vi "Build stringplusnum substring.vi"(1 "Sequence":u16(ring) items=["String1String2String3Value1Value2", "String1String2Value1String3Value2"], 2 "String1":string[](array[string]), 3 "String2":string[](array[string]), 4 "String3":string[](array[string]), 5 "error in":errorcluster, 6 "Value1":dbl[](array[numeric]) format="%.6f", 7 "Value2":dbl[](array[numeric]) format="%.6f", 8 "No.of digits Val1":i16=6, 9 "No.of digits Val2":i16=6, 10 "Input selection":T1={"With string1?"=TRUE, "With string2?"=TRUE, "With string3?"=TRUE, "With value1?"=TRUE, "With value2?"=FALSE}) -> (14 "Substring":string, 19 "error out":errorcluster)   [LabVIEW 2020]
doc: "This VI builds a command substring by combining up to three strings and two values. Sub-VI for FCG.vi, CTC.vi and DAS.vi"
panel:
  # "This vi builds a command substring by combining up to three strings and two values."
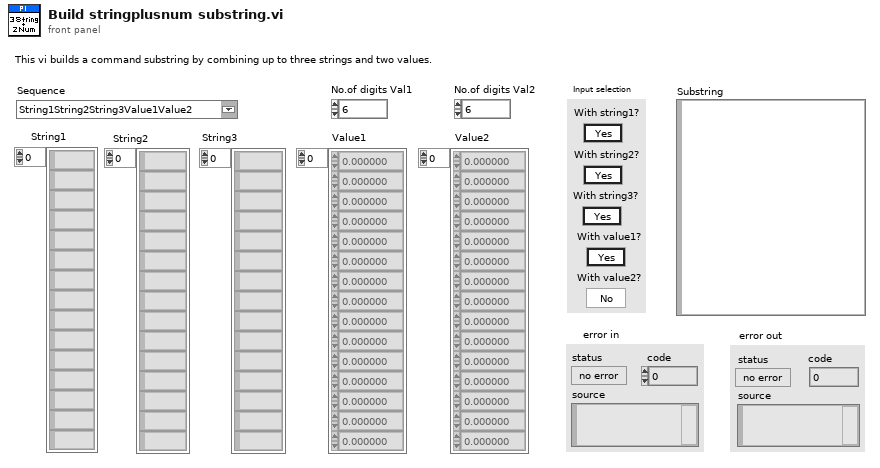
[diagram p1: front panel]
types:
  T1 = cluster{"With string1?":bool, "With string2?":bool, "With string3?":bool, "With value1?":bool, "With value2?":bool}
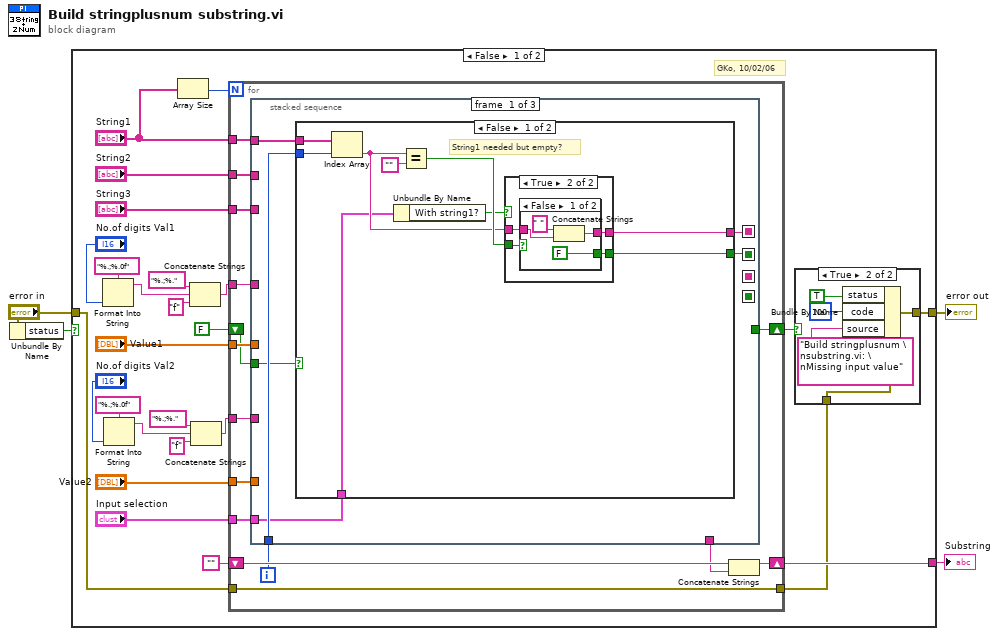
[diagram p0: block diagram]
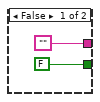
[diagram p3: hidden frame]
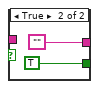
[diagram p4: hidden frame]
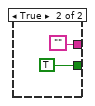
[diagram p5: hidden frame]
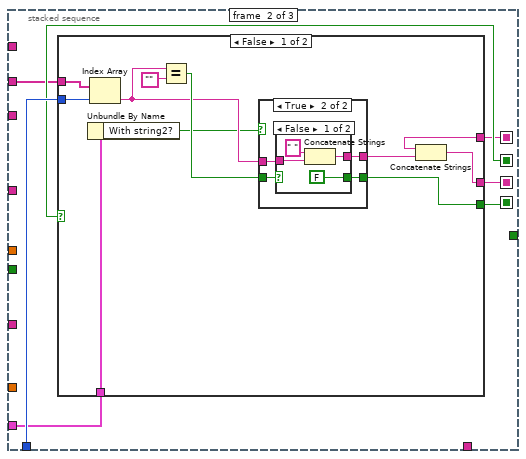
[diagram p6: hidden frame]
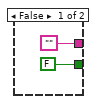
[diagram p7: hidden frame]
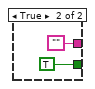
[diagram p8: hidden frame]
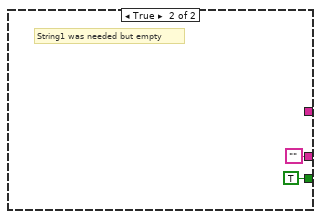
[diagram p9: hidden frame]
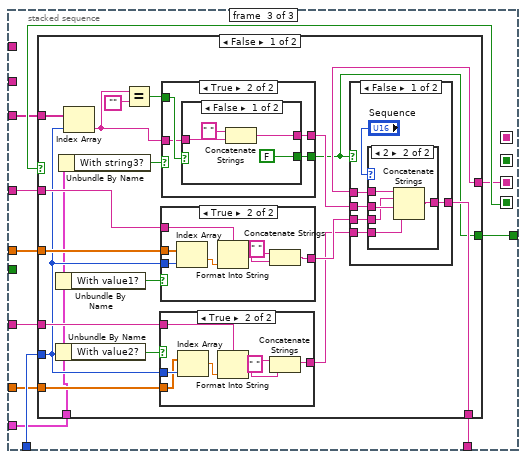
[diagram p10: hidden frame]
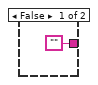
[diagram p11: hidden frame]
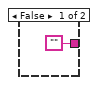
[diagram p12: hidden frame]
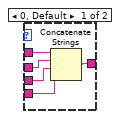
[diagram p13: hidden frame]
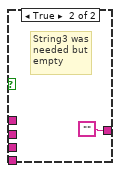
[diagram p14: hidden frame]
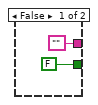
[diagram p15: hidden frame]
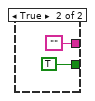
[diagram p16: hidden frame]
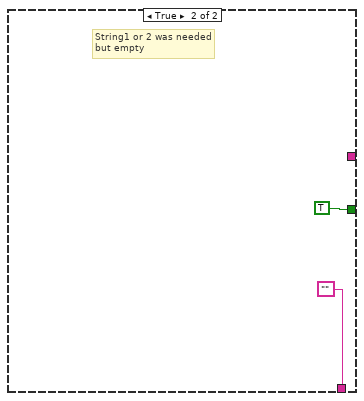
[diagram p17: hidden frame]
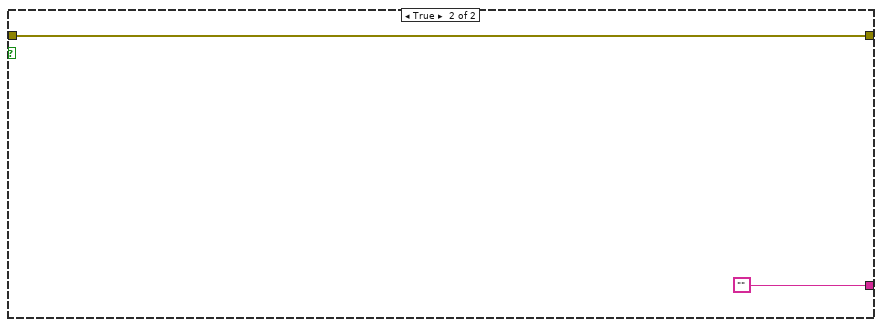
[diagram p18: hidden frame]
diagram:
  n1 = Unbundle By Name("error in") -> ("status"=w3:bool)
  n2 = case shown="False" w3 {
    tunnel: [w30 ""] -> w4
    tunnel: "error in" -> [w21 w190]
    tunnel: [w18 w190] -> w1
    frame False {
      # "GKo, 10/02/06"
      n3 = Format Into String(format string="%.;%.0f" ("Format String"), "No.of digits Val1") -> (resulting string=w13:string)  [unwired: 2 in, 1 out]
      n4 = Format Into String(format string="%.;%.0f" ("Format String"), "No.of digits Val2") -> (resulting string=w7:string)  [unwired: 2 in, 1 out]
      n5 = Array Size(array="String1") -> (size(s)=w28:i32)
      n6 = Concatenate Strings("%.;%." ("Format String"), w13, "f" ("Format String")) -> (w12:string)
      n7 = Concatenate Strings("%.;%." ("Format String"), w7, "f" ("Format String")) -> (w6:string)
      n8 = for {
        N: w28 -> [_]
        shift-right: [w50] -> w30
        shift-left: "" -> [w51]
        tunnel: "String1" -> [w48]
        tunnel: "String2" -> [w47]
        tunnel: "Value1" -> [w46]
        tunnel: w6 -> [w45]
        tunnel: "String3" -> [w44]
        tunnel: w12 -> [w42]
        tunnel: "Value2" -> [w41]
        shift-right: [w40] -> w20
        shift-left: FALSE -> [w39]
        tunnel: [w38] -> w19
        tunnel: w21 -> [w38]
        tunnel: "Input selection" -> [w37]
        i -> [w49]
        n9 = stacked-sequence {
          seq-local: [w55 _ _] -> [_ w82 _]
          seq-local: [w54 _ _] -> [_ w86 _]
          seq-local: [_ w85 _] -> [_ _ w120]
          seq-local: [_ w83 _] -> [_ _ w123]
          tunnel: w49 -> [w57 w87 w116]
          tunnel: w48 -> [w56 _ _]
          tunnel: w47 -> [_ w84 _]
          tunnel: w46 -> [_ _ w118]
          tunnel: w45 -> [_ _ w117]
          tunnel: w44 -> [_ _ w122]
          tunnel: [_ _ w121] -> w43
          tunnel: w42 -> [_ _ w119]
          tunnel: w41 -> [_ _ w115]
          tunnel: [_ _ w114] -> w40
          tunnel: w39 -> [w53 _ _]
          tunnel: w37 -> [w52 w81 w113]
          frame #0 {
            n10 = case shown="False" w53 {
              tunnel: w57 -> [w66 _]
              tunnel: w56 -> [w65 _]
              tunnel: [w61 ""] -> w55
              tunnel: [w60 TRUE] -> w54
              tunnel: w52 -> [w59 _]
              frame False {
                # "String1 needed but empty?"
                n11 = Index Array(array=w65, index=w66) -> (element=w62:string)
                n12 = Unbundle By Name(w59) -> ("With string1?"=w58:bool)
                n13 = Equal?(x=w62, y="") -> (x = y?=w63:bool)
                n14 = case shown="True" w58 {
                  tunnel: w63 -> [_ w72]
                  tunnel: ["" w71] -> w61
                  tunnel: [FALSE w70] -> w60
                  tunnel: w62 -> [_ w69]
                  frame False {
                  }
                  frame True {
                    n15 = case shown="False" w72 {
                      tunnel: [w73 ""] -> w71
                      tunnel: [FALSE TRUE] -> w70
                      tunnel: w69 -> [w75 _]
                      frame False {
                        n16 = Concatenate Strings(" " ("Substring"), w75) -> (w73:string)
                      }
                      frame True {
                      }
                    }
                  }
                }
              }
              frame True {
              }
            }
          }
          frame #1 {
            n17 = case shown="False" w86 {
              tunnel: w87 -> [w98 _]
              tunnel: [w92 ""] -> w85
              tunnel: w84 -> [w96 _]
              tunnel: [w93 TRUE] -> w83
              tunnel: w82 -> [w90 _]
              tunnel: w81 -> [w89 _]
              frame False {
                n18 = Unbundle By Name(w89) -> ("With string2?"=w88:bool)
                n19 = Index Array(array=w96, index=w98) -> (element=w94:string)
                n20 = Equal?(x=w94, y="") -> (x = y?=w95:bool)
                n21 = case shown="True" w88 {
                  tunnel: w95 -> [_ w104]
                  tunnel: ["" w103] -> w91
                  tunnel: [FALSE w102] -> w93
                  tunnel: w94 -> [_ w101]
                  frame False {
                  }
                  frame True {
                    n22 = case shown="False" w104 {
                      tunnel: [w107 ""] -> w103
                      tunnel: [FALSE TRUE] -> w102
                      tunnel: w101 -> [w105 _]
                      frame False {
                        n23 = Concatenate Strings(" " ("Substring"), w105) -> (w107:string)
                      }
                      frame True {
                      }
                    }
                  }
                }
                n24 = Concatenate Strings(w90, w91) -> (w92:string)
              }
              frame True {
                # "String1 was needed but empty"
              }
            }
          }
          frame #2 {
            n25 = case shown="False" w123 {
              tunnel: [w138 ""] -> w121
              tunnel: w122 -> [w142 _]
              tunnel: w120 -> [w125 _]
              tunnel: w119 -> [w136 _]
              tunnel: w118 -> [w135 _]
              tunnel: w117 -> [w134 _]
              tunnel: w116 -> [w133 _]
              tunnel: w115 -> [w132 _]
              tunnel: [w124 TRUE] -> w114
              tunnel: w113 -> [w129 _]
              frame False {
                n26 = Unbundle By Name(w129) -> ("With value1?"=w127:bool)
                n27 = Unbundle By Name(w129) -> ("With value2?"=w126:bool)
                n28 = Unbundle By Name(w129) -> ("With string3?"=w128:bool)
                n29 = Index Array(array=w142, index=w133) -> (element=w139:string)
                n30 = Equal?(x=w139, y="") -> (x = y?=w140:bool)
                n31 = case shown="True" w126 {
                  tunnel: w134 -> [_ w147]
                  tunnel: w133 -> [_ w146]
                  tunnel: ["" w145] -> w130
                  tunnel: w132 -> [_ w144]
                  frame False {
                  }
                  frame True {
                    n32 = Index Array(array=w144, index=w146) -> (element=w150:dbl)
                    n33 = Format Into String(format string=w147, w150) -> (resulting string=w148:string)  [unwired: 2 in, 1 out]
                    n34 = Concatenate Strings(" " ("Substring"), w148) -> (w145:string)
                  }
                }
                n35 = case shown="True" w127 {
                  tunnel: w136 -> [_ w155]
                  tunnel: w133 -> [_ w154]
                  tunnel: ["" w153] -> w131
                  tunnel: w135 -> [_ w152]
                  frame False {
                  }
                  frame True {
                    n36 = Index Array(array=w152, index=w154) -> (element=w158:dbl)
                    n37 = Format Into String(format string=w155, w158) -> (resulting string=w156:string)  [unwired: 2 in, 1 out]
                    n38 = Concatenate Strings(" " ("Substring"), w156) -> (w153:string)
                  }
                }
                n39 = case shown="True" w128 {
                  tunnel: w140 -> [_ w181]
                  tunnel: ["" w180] -> w137
                  tunnel: [FALSE w179] -> w124
                  tunnel: w139 -> [_ w178]
                  frame False {
                  }
                  frame True {
                    n40 = case shown="False" w181 {
                      tunnel: [w184 ""] -> w180
                      tunnel: [FALSE TRUE] -> w179
                      tunnel: w178 -> [w182 _]
                      frame False {
                        n41 = Concatenate Strings(" " ("Substring"), w182) -> (w184:string)
                      }
                      frame True {
                      }
                    }
                  }
                }
                n42 = case shown="False" w124 {
                  tunnel: [w163 ""] -> w138
                  tunnel: w125 -> [w162 _]
                  tunnel: w137 -> [w161 _]
                  tunnel: w131 -> [w160 _]
                  tunnel: w130 -> [w159 _]
                  frame False {
                    n43 = case shown="2" "Sequence" {
                      tunnel: [w169 w174] -> w163
                      tunnel: w162 -> [w168 w173]
                      tunnel: w161 -> [w167 w172]
                      tunnel: w160 -> [w166 w171]
                      tunnel: w159 -> [w165 w170]
                      frame 0, Default {
                        n44 = Concatenate Strings(w168, w167, w166, w165) -> (w169:string)
                      }
                      frame 2 {
                        n45 = Concatenate Strings(w173, w171, w172, w170) -> (w174:string)
                      }
                    }
                  }
                  frame True {
                    # "String3 was\nneeded but\nempty"
                  }
                }
              }
              frame True {
                # "String1 or 2 was needed\nbut empty"
              }
            }
          }
        }
        n46 = Concatenate Strings(w51, w43) -> (w50:string)
      }
      n47 = case shown="True" w20 {
        tunnel: [w31 w33] -> w18
        tunnel: w19 -> [w31 w34]
        frame False {
        }
        frame True {
          n48 = Bundle By Name(cluster=w34, "status"=TRUE, "code"=100, "source"="Build stringplusnum \nsubstring.vi: \nMissing input value") -> (w33:errorcluster)
        }
      }
    }
    frame True {
    }
  }
  "Substring" <- w4
  "error out" <- w1
